vi "Date and Time Filter Data.vi"(8 "error in (no error)":errorcluster, 9 "Stop Time Stamp":timestamp format="%<%x %.3X>T", 10 "Start Time Stamp":timestamp format="%<%x %.3X>T", 11 "FE FF Frame in":refnum<class "FE FF Frame.lvclass">) -> (0 "error out":errorcluster, 3 "FE FF Frame out":refnum<class "FE FF Frame.lvclass">)   [LabVIEW 2023, in "Data Analysis.lvlib" / "FE FF Frame.lvlib" / "FE FF Frame.lvclass"]
uses:
  FE FF Frame.lvclass
  <vilib>/Utility/miscctls.llb/LVRowAndColumnUnsignedTypeDef.ctl
  FE FF Frame.lvclass/FE FF Frame.ctl
  HardwareAbstractionLayer_LVOOP/Database/Database.lvclass
  Data Analysis.lvlib
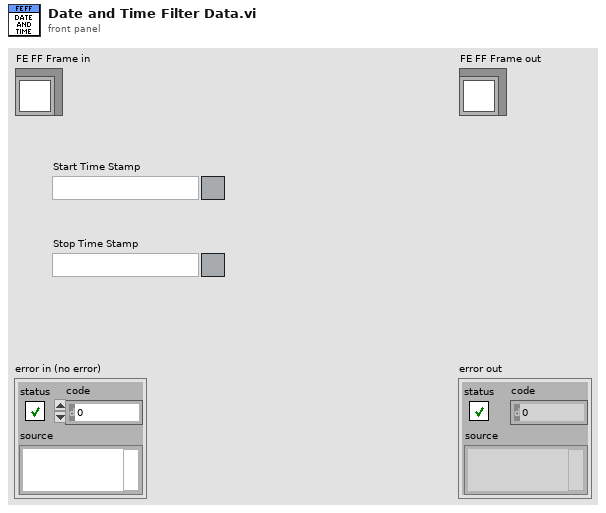
[diagram p1: front panel]
types:
  T1 = typedef "LVRowAndColumnUnsignedTypeDef.ctl" = cluster{"Row":u32, "Column":u32}
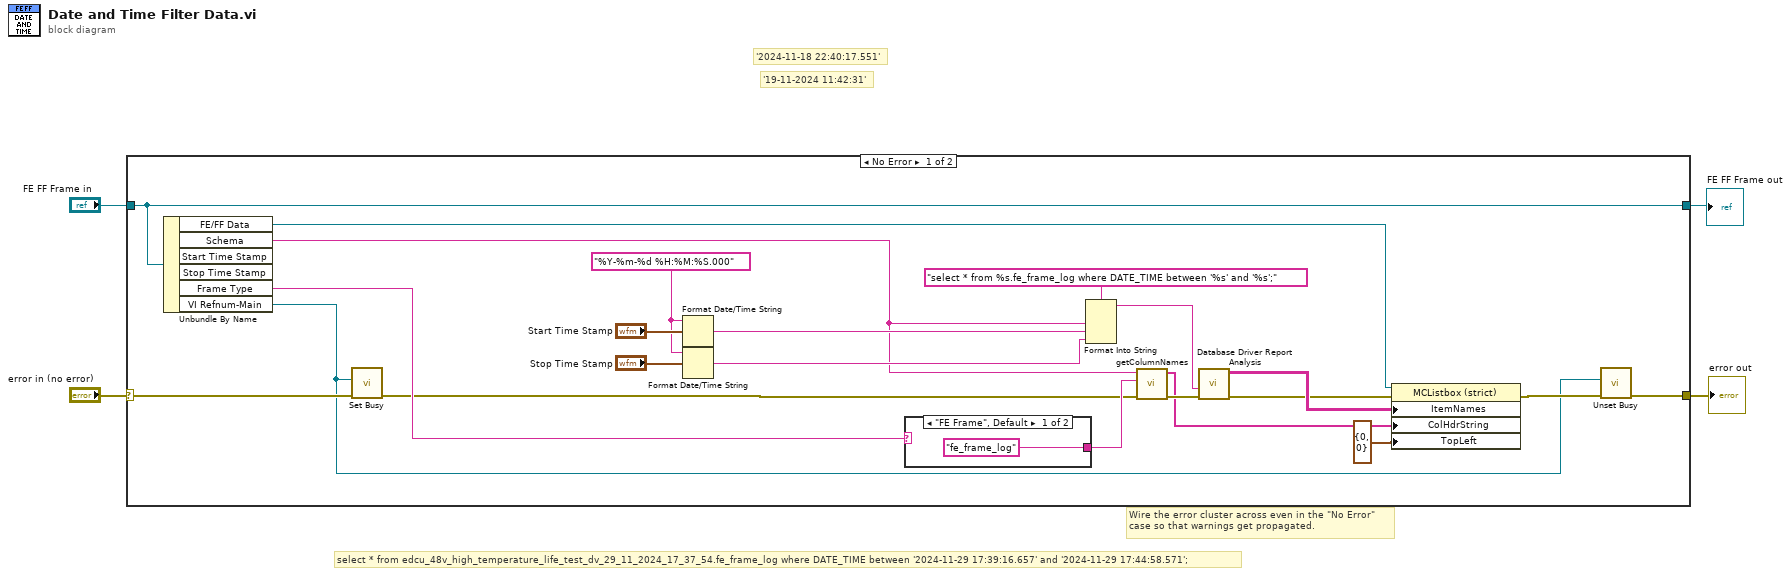
[diagram p0: block diagram]
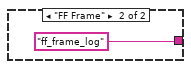
[diagram p2: hidden frame]
diagram:
  # "'19-11-2024 11:42:31'"
  # "'2024-11-18 22:40:17.551'"
  # "Wire the error cluster across even in the \"No Error\"\ncase so that warnings get propagated."
  # "select * from edcu_48v_high_temperature_life_test_dv_29_11_2024_17_37_54.fe_frame_log where DATE_TIME between '2024-11-29 17:39:16.657' and '2024-11-29 17:44:58.571';"
  n1 = case shown="No Error" "error in (no error)" {
    selector: "error in (no error)" -> [w9 w30]
    tunnel: [w7 w30] -> w3
    tunnel: [w26 w29] -> w1
    tunnel: "FE FF Frame in" -> [w26 w29]
    frame No Error {
      w5 = "%Y-%m-%d %H:%M:%S.000" ("time format string (%c)")
      n2 = Unbundle By Name(w26) -> ("FE/FF Data"=w23:refnum<vi>, "Schema"=w17:string, "Frame Type"=w14:string, "VI Refnum-Main"=w6:refnum<vi>)  [unwired: 2 out]
      n3 = call <vilib>:"Set Busy.vi"("error in (no error)"=w9, "VI reference (current VI)"=w6) -> ("error out"=w8:errorcluster)  [unwired: 8 in, 1 out]
      n4 = Format Date/Time String(time format string (%c)=w5, seconds (now)="Start Time Stamp") -> (date/time string=w19:string)  [unwired: 1 in]
      n5 = Format Date/Time String(time format string (%c)=w5, seconds (now)="Stop Time Stamp") -> (date/time string=w18:string)  [unwired: 1 in]
      n6 = case shown="\"FE Frame\", Default" w14 {
        tunnel: ["fe_frame_log" "ff_frame_log"] -> w13
        frame "FE Frame", Default {
        }
        frame "FF Frame" {
        }
      }
      n7 = Format Into String(format string="select * from %s.fe_frame_log where DATE_TIME between '%s' and '%s';", w17, w19, w18) -> (resulting string=w20:string)  [unwired: 2 in, 1 out]
      n8 = call "getColumnNames.vi"("error in (no error)"=w8, "tableName"=w13, "schema"=w17) -> ("error out"=w16:errorcluster, "columnNames"=w15:string[])  [unwired: 6 in, 1 out]
      n9 = call "Database Driver Report Analysis.vi"("error in"=w16, "SQL query"=w20) -> ("error out"=w24:errorcluster, "data"=w25:string[][])  [unwired: 6 in, 2 out]
      n10 = property class="MCListbox (strict)"(reference=w23, error in=w24, "ItemNames"=w25, "ColHdrString"=w15, "TopLeft"=T1 {"Row"=0, "Column"=0} ("Top Left Visible Cell")) -> (error out=w22:errorcluster)  [unwired: 1 out]
      n11 = call <vilib>:"Unset Busy.vi"("error in (no error)"=w22, "VI reference (current VI)"=w6) -> ("error out"=w7:errorcluster)  [unwired: 9 in]
    }
    frame Error {
    }
  }
  "error out" <- w3
  "FE FF Frame out" <- w1
